vi "Read Key Value Path.vi"(7 "Section Name":string, 8 "error in (no error)":errorcluster, 9 "Default":path, 10 "Key Name":string, 11 "ODBC-Interface in":refnum<class "ODBC-Interface.lvclass">) -> (0 "error out":errorcluster, 1 "Value":path, 2 "found":bool, 3 "ODBC-Interface out":refnum<class "ODBC-Interface.lvclass">)   [LabVIEW 2016, in "DB-Configuration.lvlib" / "ODBC-Interface.lvclass"]
doc: "Read path key value."
uses:
  ODBC-Interface.lvclass
  <vilib>/addons/database/_DB Variant To Data/Database Variant To Data.xnode
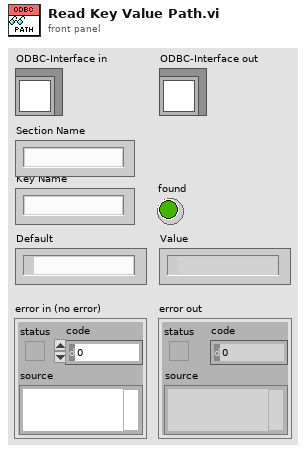
[diagram p1: front panel]
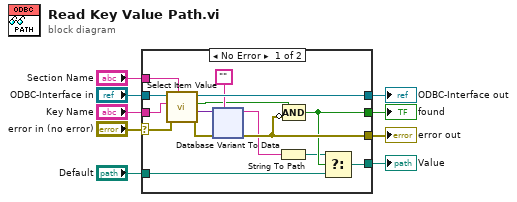
[diagram p0: block diagram]
diagram:
  n1 = case shown="No Error" "error in (no error)" {
    selector: "error in (no error)" -> [w12 w58]
    tunnel: "ODBC-Interface in" -> [w24 w59]
    tunnel: [w23 w59] -> w4
    tunnel: "Section Name" -> [w22 _]
    tunnel: "Key Name" -> [w21 _]
    tunnel: [w16 w58] -> w2
    tunnel: [w15 _] -> w3
    tunnel: [w14 w57] -> w1
    tunnel: "Default" -> [w13 w57]
    frame No Error {
      n2 = call-dynamic "Select Item Value.vi"("Section Name"=w22, "error in (no error)"=w12, "Key Name"=w21, "ODBC-Interface in"=w24) -> ("error out"=w19:errorcluster, "Value"=w20:variant, "found"=w17:bool, "ODBC-Interface out"=w23:refnum<class "ODBC-Interface.lvclass">)  [unwired: 4 in]
      n3 = xnode "Database Variant To Data"("database variant"=w20, "error in (no error)"=w19, "type"="") -> ("data"=w11:string, "error out"=w16:errorcluster)
      n4 = String To Path(string=w11) -> (path=w10:path)
      n5 = Compound Arithmetic op=AND(w17, invert w16) -> (w15:bool)
      n6 = Select(t=w10, s=w15, f=w13) -> (s? t:f=w14:path)
    }
    frame Error {
    }
  }
  "error out" <- w2
  "ODBC-Interface out" <- w4
  "Value" <- w1
  "found" <- w3
